vi "AT+TT.vi"(8 "错误输入（无错误）":errorcluster, 10 "Count":i32=2, 11 "站号":u16) -> (0 "错误输出":errorcluster, 3 "FIND?":bool)   [LabVIEW 2016, in "斯坦道原位多参数.lvlib"]
uses:
  <vilib>/Plasmionique/MB Master/MB_Master_Serial/MB_Master_Serial.lvclass/MB_Master_Serial.ctl
  <vilib>/Plasmionique/MB Master/MB_Master_Serial/Read VISA Resource.vi
  <vilib>/Plasmionique/MB Master/MB_VISA_Lock/MB_VISA_Lock.lvlib
  <vilib>/Plasmionique/MB Master/MB_Master_Serial/MB_Master_Serial.lvclass
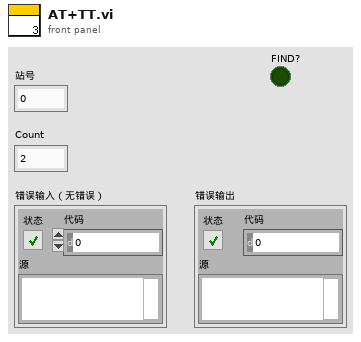
[diagram p1: front panel]
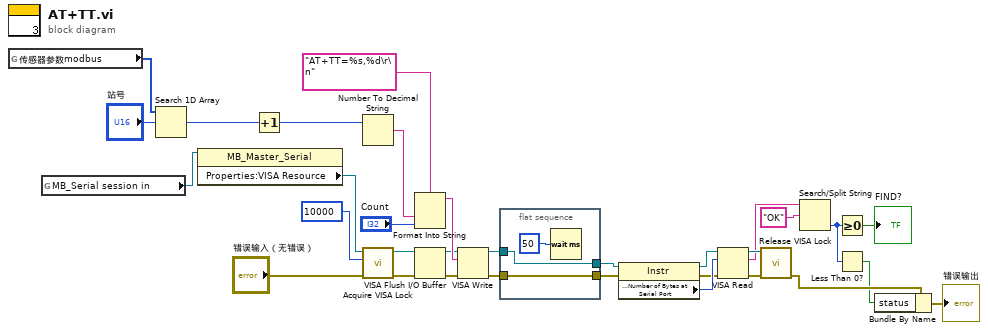
[diagram p0: block diagram]
diagram:
  n1 = global read "多参数断电保存全局变量.vi" "传感器参数modbus"() -> (w25:u16[])
  n2 = global read "多参数全局变量.vi" "MB_Serial session in"() -> (w23:refnum<class "MB_Master_Serial.lvclass">)
  n3 = Search 1D Array(1D array=w25, element="站号") -> (index of element=w31:i32)  [unwired: 1 in]
  n4 = property class="MB_Master_Serial"(reference=w23) -> ("Properties:VISA Resource"=w21:refnum<visa-resource-name>)  [unwired: 1 in, 2 out]
  n5 = Increment(x=w31) -> (x+1=w32:i32)
  n6 = Number To Decimal String(number=w32) -> (decimal integer string=w26:string)  [unwired: 1 in]
  n7 = call <vilib>:"Acquire VISA Lock.vi"("error in (no error)"="错误输入（无错误）", "timeout in ms (-1)"=10000, "VISA resource name"=w21) -> ("error out"=w19:errorcluster, "VISA resource name out"=w20:refnum<visa-resource-name>)  [unwired: 7 in]
  n8 = Format Into String(format string="AT+TT=%s,%d\r\n" ("写入缓冲区"), w26, "Count") -> (resulting string=w27:string)  [unwired: 2 in, 1 out]
  n9 = VISA Flush I/O Buffer(VISA resource name=w20, error in (no error)=w19) -> (VISA resource name out=w18:refnum<visa-resource-name>, error out=w17:errorcluster)  [unwired: 1 in]
  n10 = VISA Write(VISA resource name=w18, write buffer=w27, error in (no error)=w17) -> (VISA resource name out=w13:refnum<visa-resource-name>, error out=w12:errorcluster)  [unwired: 1 out]
  n11 = flat-sequence {
    tunnel: w13 -> [w34]
    tunnel: [w35] -> w8
    tunnel: w12 -> [w35]
    tunnel: [w34] -> w11
    frame #0 {
      n12 = Wait (ms)(milliseconds to wait=u32 50 ("等待时间（毫秒）")) -> ()  [unwired: 1 out]
    }
  }
  n13 = property class="Instr"(reference=w11, error in=w8) -> (reference out=w9:refnum<visa-resource-name>, error out=w7:errorcluster, "Serial Settings:Number of Bytes at Serial Port"=w10:u32)
  n14 = VISA Read(VISA resource name=w9, byte count=w10, error in (no error)=w7) -> (VISA resource name out=w15:refnum<visa-resource-name>, read buffer=w6:string, error out=w14:errorcluster)  [unwired: 1 out]
  n15 = call <vilib>:"Release VISA Lock.vi"("error in (no error)"=w14, "VISA resource name"=w15) -> ("error out"=w30:errorcluster)  [unwired: 8 in, 1 out]
  n16 = Search/Split String(string=w6, search string/char (-)="OK" ("搜索字符串/字符(-)")) -> (offset of match=w2:i32)  [unwired: 1 in, 2 out]
  n17 = Greater Or Equal To 0?(x=w2) -> (x >= 0?=→"FIND?":bool)
  n18 = Less Than 0?(x=w2) -> (x < 0?=w1:bool)
  n19 = Bundle By Name(cluster=w30, "status"=w1) -> (→"错误输出":errorcluster)
